vi "Read Multiple.vi"(7 "timeout in ms (-1)":i32=-1, 9 "number to read (-1, available)":i32=-1, 10 "channel":T1) -> (1 "last element?":bool, 2 "elements":T2[](array[typedef]), 5 "timed out?":bool, 6 "count":i32)   [LabVIEW 2017, in "Stream-t'WPI_EncoderType.ctl'.lvlib"]
doc: "Reads multiple elements as a block from a Stream channel. You can configure how and when the channel waits for multiple elements."
uses:
  <extravilib>/ChannelInstances/Stream-t'WPI_EncoderType.ctl'.lvlib
  <vilib>/Rock Robotics/WPI/Encoder/WPI_EncoderType.ctl
  <extravilib>/ChannelInstances/Stream-t'WPI_EncoderType.ctl'/)Channel.ctl
  <extravilib>/ChannelInstances/Stream-t'WPI_EncoderType.ctl'/Read With Abort.vi
  <extravilib>/ChannelInstances/Stream-t'WPI_EncoderType.ctl'/EndpointRead.vi
  <resource>/ChannelSupport/_ChannelSupport/WaitIfNeeded.vi
  <extravilib>/ChannelInstances/Stream-t'WPI_EncoderType.ctl'/)Channel.vi
  <resource>/ChannelSupport/_ChannelSupport/GetErrors/FpgaChannelWireNotSupported.xnode
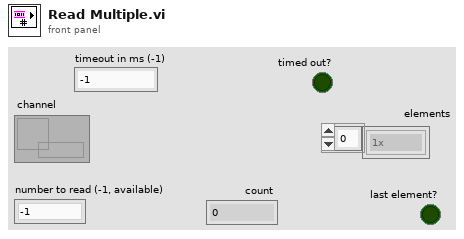
[diagram p1: front panel]
types:
  T1 = typedef "Stream-t'WPI_EncoderType.ctl'.lvlib/)Channel.ctl" = refnum<queue>
  T2 = typedef "WPI_EncoderType.ctl" = enum16{"1x", "2x", "4x"}
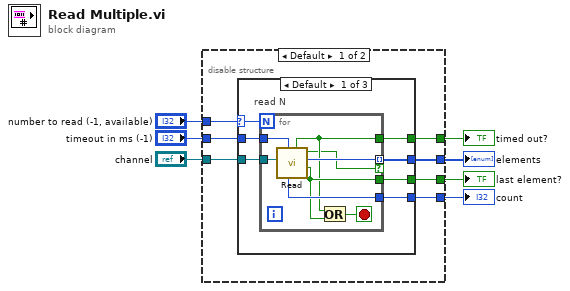
[diagram p0: block diagram]
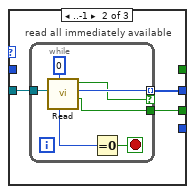
[diagram p2: hidden frame]
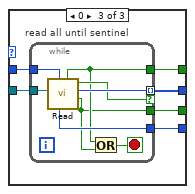
[diagram p3: hidden frame]
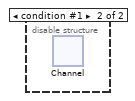
[diagram p4: hidden frame]
diagram:
  n1 = disable-structure shown="Default" {
    disable-tunnel: "channel" -> [w14 _]
    disable-tunnel: [w13 _] -> w6
    disable-tunnel: [w12 _] -> w5
    disable-tunnel: "number to read (-1, available)" -> [w11 _]
    disable-tunnel: [w10 _] -> w3
    disable-tunnel: "timeout in ms (-1)" -> [w9 _]
    disable-tunnel: [w8 _] -> w1
    frame condition #0 (active) {
      n2 = case shown="Default" w11 {
        selector: w11 -> [w18 _ _]
        tunnel: w14 -> [w21 w32 w45]
        tunnel: [w20 w31 w44] -> w13
        tunnel: [w19 _ w43] -> w12
        tunnel: [w15 w30 w40] -> w10
        tunnel: w9 -> [w17 _ w42]
        tunnel: [w16 _ w41] -> w8
        frame Default {
          # "read N"
          n3 = for {
            N: w18 -> [_]
            tunnel: w21 -> [w29]
            tunnel: [w28] -> w20 mode=indexing if=w22
            tunnel: [w27] -> w19
            tunnel: w17 -> [w26]
            tunnel: [w24] -> w16
            tunnel: [w25] -> w15
            stop <- w23 stop-if-true
            n4 = call <extravilib>:"Read.vi"("timeout in ms (-1)"=w26, "channel"=w29) -> ("last element?"=w25:bool, "element"=w28:T2, "element valid?"=w22:bool, "timed out?"=w24:bool, "count"=w27:i32)  [unwired: 5 in]
            n5 = Or(x=w24, y=w25) -> (x .or. y?=w23:bool)
          }
        }
        frame ..-1 {
          # "read all immediately available"
          n6 = while {
            tunnel: w32 -> [w38]
            tunnel: [w37] -> w31 mode=indexing if=w35
            tunnel: [w33] -> w30
            stop <- w39 stop-if-true
            n7 = call <extravilib>:"Read.vi"("timeout in ms (-1)"=0, "channel"=w38) -> ("last element?"=w33:bool, "element"=w37:T2, "element valid?"=w35:bool, "count"=w36:i32)  [unwired: 5 in, 1 out]
            n8 = Equal To 0?(x=w36) -> (x = 0?=w39:bool)
          }
        }
        frame 0 {
          # "read all until sentinel"
          n9 = while {
            tunnel: w45 -> [w53]
            tunnel: [w52] -> w44 mode=indexing if=w49
            tunnel: [w51] -> w43
            tunnel: w42 -> [w50]
            tunnel: [w47] -> w41
            tunnel: [w46] -> w40
            stop <- w48 stop-if-true
            n10 = call <extravilib>:"Read.vi"("timeout in ms (-1)"=w50, "channel"=w53) -> ("last element?"=w46:bool, "element"=w52:T2, "element valid?"=w49:bool, "timed out?"=w47:bool, "count"=w51:i32)  [unwired: 5 in]
            n11 = Or(x=w47, y=w46) -> (x .or. y?=w48:bool)
          }
        }
      }
    }
    frame condition #1 {
      n12 = xnode "Channel"() -> ()
    }
  }
  "elements" <- w6
  "count" <- w5
  "timed out?" <- w1
  "last element?" <- w3
